vi "testPsuBasic.vi"() -> ()   [LabVIEW 2023]
doc: "Debugging and testing of power supply abstraction."
uses:
  Data/PsuTypes.ctl
  9f57c3dc-461e-4f3e-a001-c2da2c6ac9e6.vi
  PowerSupply.lvclass
  swePsu.lvlib
panel:
  out "error out":errorcluster
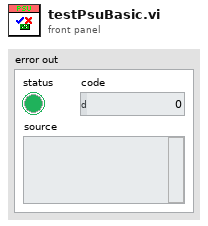
[diagram p1: front panel]
types:
  T1 = typedef "swePsu.lvlib/PsuTypes.ctl" = enum16{"Simulated", "PSU_NI", "PSU_TTi"}
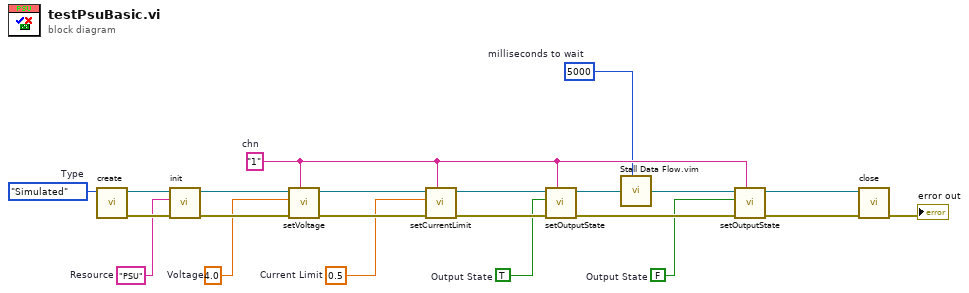
[diagram p0: block diagram]
diagram:
  w2 = PsuTypes."Simulated"  # Type
  w3 = "PSU"  # Resource
  w4 = 4.0  # Voltage
  w5 = 0.5  # Current Limit
  w6 = TRUE  # Output State
  w7 = u32 5000  # milliseconds to wait
  w8 = FALSE  # Output State
  w9 = "1"  # chn
  n1 = call "create.vi"("Type"=w2) -> ("error out"=w21:errorcluster, "PowerSupply.lvclass"=w22:refnum<class "PowerSupply.lvclass">)  [unwired: 9 in]
  n2 = call-dynamic "init.vi"("error in (no error)"=w21, "Resource"=w3, "Instrument in"=w22) -> ("error out"=w19:errorcluster, "Instrument out"=w20:refnum<class "PowerSupply.lvclass">)  [unwired: 7 in]
  n3 = call-dynamic "setVoltage.vi"("chn"=w9, "error in (no error)"=w19, "Voltage"=w4, "PowerSupply in"=w20) -> ("error out"=w17:errorcluster, "PowerSupply out"=w18:refnum<class "PowerSupply.lvclass">)  [unwired: 6 in]
  n4 = call-dynamic "setCurrentLimit.vi"("chn"=w9, "error in (no error)"=w17, "Current Limit"=w5, "PowerSupply in"=w18) -> ("error out"=w15:errorcluster, "PowerSupply out"=w16:refnum<class "PowerSupply.lvclass">)  [unwired: 6 in]
  n5 = call-dynamic "setOutputState.vi"("chn"=w9, "error in (no error)"=w15, "Output State"=w6, "PowerSupply in"=w16) -> ("error out"=w12:errorcluster, "PowerSupply out"=w14:refnum<class "PowerSupply.lvclass">)  [unwired: 6 in]
  n6 = call "Stall Data Flow.vim"("value in"=w14, "milliseconds to wait"=w7) -> ("value out"=w13:refnum<class "PowerSupply.lvclass">)  [unwired: 1 out]
  n7 = call-dynamic "setOutputState.vi"("chn"=w9, "error in (no error)"=w12, "Output State"=w8, "PowerSupply in"=w13) -> ("error out"=w10:errorcluster, "PowerSupply out"=w11:refnum<class "PowerSupply.lvclass">)  [unwired: 6 in]
  n8 = call-dynamic "close.vi"("error in (no error)"=w10, "Instrument in"=w11) -> ("error out"=→"error out":errorcluster)  [unwired: 9 in]
